vi "rwfm_AcqRead(Wfm).vi"(6 "Timeout (s)":dbl=5.0, 7 "Poll Time (ms)":u32=10, 8 "error in":errorcluster, 9 "Samps Read per Chan":i32, 10 "Sampling Info":T2={"Number of Channels"=4, "Sampling Rate"=5120.0, "Channels"=[], "Units"=[], "Offsets"=[]}, 11 "Dynamic FPGA VI Reference":T1) -> (0 "error out":errorcluster, 1 "Samples Remaining":u32, 2 "Wfm Data":waveform(sgl)[](array[waveform]), 3 "Dynamic FPGA VI Reference":T1, 4 "Data Rate [S/s]":u32, 5 "Time Stamp":timestamp)   [LabVIEW 2017, in "cRIOWfmLib.lvlib"]
doc: "Reads waveform data from the DMA FIFO."
uses:
  <vilib>/addons/InsightCM/Devices/Shared/Cms/cRIOWfmAcq/cRIOWfmLib.lvlib
  <vilib>/addons/InsightCM/Devices/Shared/Cms/cRIOWfmAcq/subVIs/RIO Wfm Cust Ctrls/rwfm_SamplingInfo.ctl
  <vilib>/addons/InsightCM/Devices/Shared/Cms/cRIOWfmAcq/subVIs/RIO Wfm Cust Ctrls/rwfm_DynamicFPGAref2.ctl
  <vilib>/Utility/error.llb/Error Cluster From Error Code.vi
  <vilib>/rvi/errors/niLvFpgaAdjustHostInterfaceError.vi
  <vilib>/rvi/interface/nirviReadWriteControl/nirviReadWriteControl.xnode
  <vilib>/rvi/interface/nirviMethod/nirviMethod.xnode
  NiFpgaLv.dll
  <vilib>/rvi/interface/Simulation/niFpgaSimulationCallBeginRW.vi
  <vilib>/FPGAPlugInAG/Dynamic/niLvFpga_ReadFifo_Dynamic.vi
  <vilib>/rvi/errors/niLvFpgaMergeErrorWithErrorCode.vi
panel:
  out "Read Time (ms)":u32
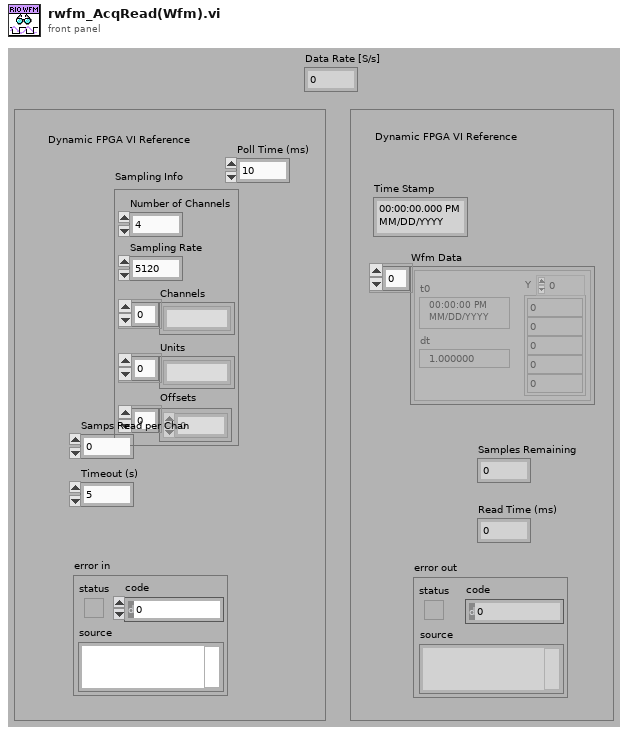
[diagram p1: front panel]
types:
  T1 = typedef "cRIOWfmLib.lvlib/rwfm_DynamicFPGAref2.ctl" = refnum<k20>
  T2 = typedef "cRIOWfmLib.lvlib/rwfm_SamplingInfo.ctl" = cluster{"Number of Channels":i32, "Sampling Rate":dbl, "Channels":string[], "Units":string[], "Offsets":sgl[]}
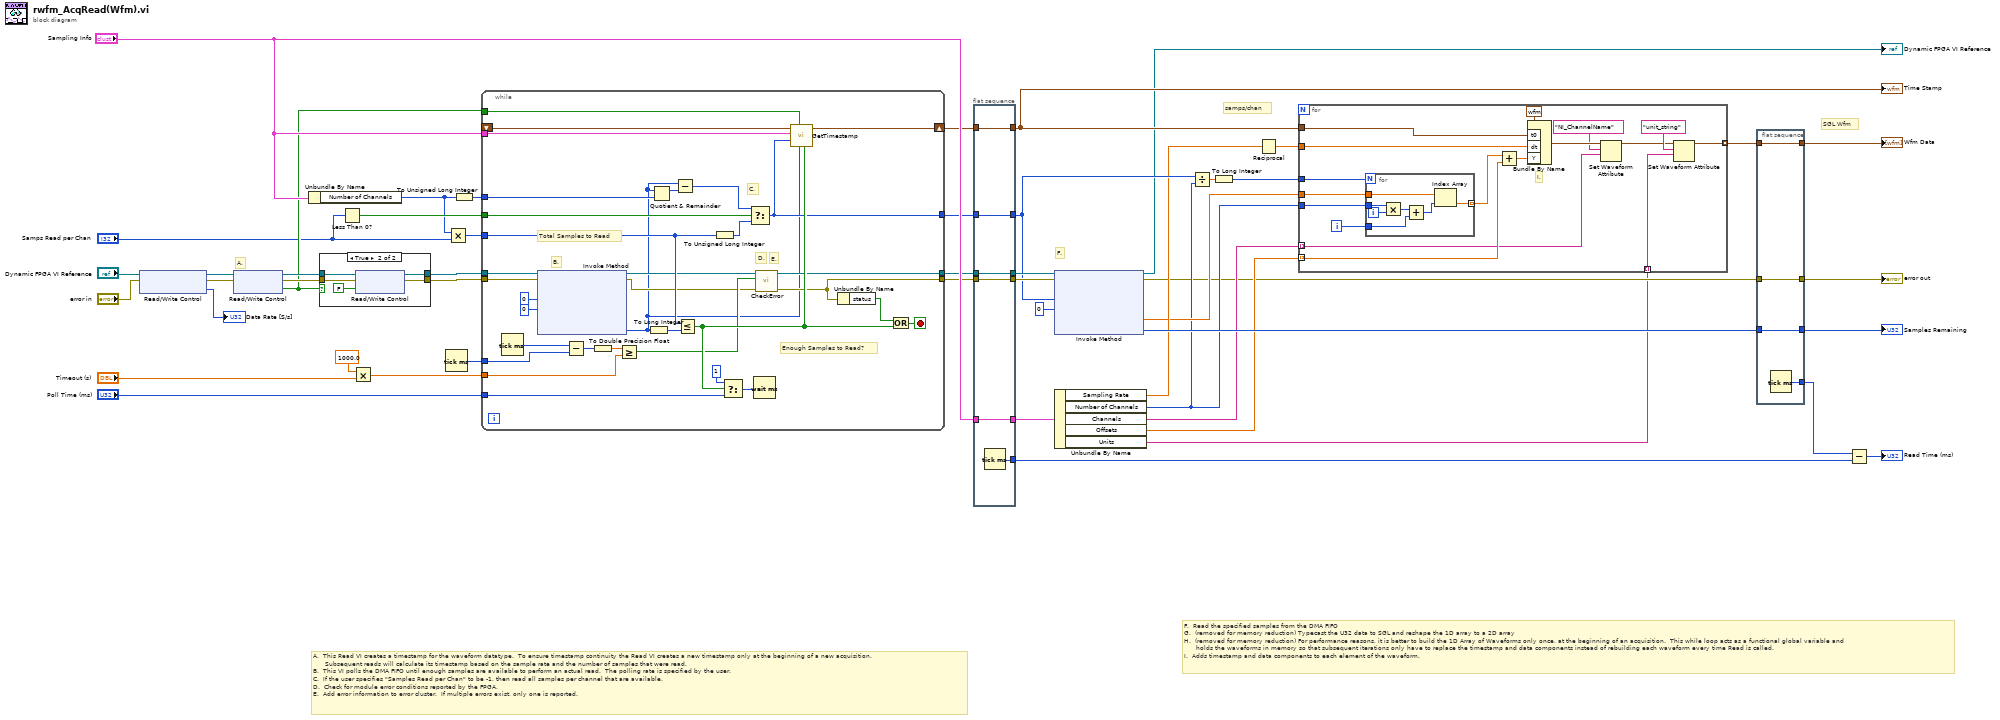
[diagram p0: block diagram]
diagram:
  # "samps/chan"
  # "SGL Wfm"
  # "F."
  # "F.  Read the specified samples from the DMA FIFO\nG.  (removed for memory reduction) Typecast the U32 data to SGL and reshape the 1D array to a 2D array\nH.  (removed for memory reduction) For performance reasons, it is better to build the 1D Array of Waveforms only once, at the beginning of an acquisition.  This while loop acts as a functional global variable and\n      holds the waveforms in memory so that subsequent iterations only have to replace the timestamp and data components instead of rebuilding each waveform every time Read is called.\nI.  Adds timestamp and data components to each element of the waveform."
  # "A.  This Read VI creates a timestamp for the waveform datatype.  To ensure timestamp continuity the Read VI creates a new timestamp only at the beginning of a new acquisition.  \n      Subsequent reads will calculate its timestamp based on the sample rate and the number of samples that were read.\nB.  This VI polls the DMA FIFO until enough samples are available to perform an actual read.  The polling rate is specified by the user.\nC.  If the user specifies \"Samples Read per Chan\" to be -1, then read all samples per channel that are available.\nD.  Check for module error conditions reported by the FPGA.\nE.  Add error information to error cluster.  If multiple errors exist, only one is reported."
  # "A."
  n1 = xnode "Read/Write Control"("FPGA VI Reference In"="Dynamic FPGA VI Reference", "error in"="error in") -> ("FPGA VI Reference Out"=w11:T1, "error out"=w14:errorcluster, "Data Rate [S/s]"=→"Data Rate [S/s]":u32)
  n2 = xnode "Read/Write Control"("FPGA VI Reference In"=w11, "error in"=w14) -> ("FPGA VI Reference Out"=w49:T1, "error out"=w50:errorcluster, "First Read"=w23:bool)
  n3 = Unbundle By Name("Sampling Info") -> ("Number of Channels"=w17:i32)
  n4 = case shown="True" w23 {
    tunnel: w49 -> [w52 w57]
    tunnel: [w52 w56] -> w48
    tunnel: w50 -> [w51 w55]
    tunnel: [w51 w54] -> w47
    frame False {
    }
    frame True {
      n5 = xnode "Read/Write Control"("FPGA VI Reference In"=w57, "error in"=w55, "First Read"=FALSE) -> ("FPGA VI Reference Out"=w56:T1, "error out"=w54:errorcluster)
    }
  }
  n6 = Less Than 0?(x="Samps Read per Chan") -> (x < 0?=w31:bool)
  n7 = Multiply(x=1000.0 ("y"), y="Timeout (s)") -> (x*y=w43:dbl)
  n8 = Tick Count (ms)() -> (millisecond timer value=w46:u32)
  n9 = Multiply(x=w17, y="Samps Read per Chan") -> (x*y=w30:i32)
  n10 = To Unsigned Long Integer(number=w17) -> (unsigned 32bit integer=w28:u32)
  n11 = while {
    tunnel: [w61] -> w34
    tunnel: [w64] -> w35
    tunnel: w23 -> [w80]
    tunnel: w48 -> [w84]
    tunnel: w47 -> [w83]
    shift-right: [w74] -> w33
    shift-left: _ -> [w81]
    tunnel: "Sampling Info" -> [w82]
    tunnel: w46 -> [w85]
    tunnel: w43 -> [w86]
    tunnel: "Poll Time (ms)" -> [w76]
    tunnel: w30 -> [w69]
    tunnel: [w67] -> w32
    tunnel: w31 -> [w72]
    tunnel: w28 -> [w68]
    stop <- w87 stop-if-true
    # "E."
    # "D."
    # "C."
    # "B."
    # "Total Samples to Read"
    # "Enough Samples to Read?"
    n12 = Tick Count (ms)() -> (millisecond timer value=w79:u32)
    n13 = xnode "Invoke Method"("FPGA VI Reference In"=w84, "error in"=w83, "Number of Elements"=u32 0, "Timeout (ms)"=0) -> ("FPGA VI Reference Out"=w63:T1, "error out"=w62:errorcluster, "Elements Remaining"=w58:u32)  [unwired: 1 out]
    n14 = Subtract(x=w79, y=w85) -> (x-y=w90:u32)
    n15 = To Double Precision Float(number=w90) -> (double precision float=w89:dbl)
    n16 = Greater Or Equal?(x=w89, y=w86) -> (x >= y?=w73:bool)
    n17 = To Long Integer(number=w58) -> (32bit integer=w71:i32)
    n18 = Quotient & Remainder(x=w58, y=w68) -> (x-y*floor(x/y)=w66:u32)  [unwired: 1 out]
    n19 = Subtract(x=w58, y=w66) -> (x-y=w65:u32)
    n20 = Less Or Equal?(x=w69, y=w71) -> (x <= y?=w78:bool)
    n21 = To Unsigned Long Integer(number=w69) -> (unsigned 32bit integer=w70:u32)
    n22 = Select(t=u32 1, s=w78, f=w76) -> (s? t:f=w77:u32)
    n23 = Select(t=w65, s=w72, f=w70) -> (s? t:f=w67:u32)
    n24 = Wait (ms)(milliseconds to wait=w77) -> ()  [unwired: 1 out]
    n25 = call <vilib>:"CheckError.vi"("error in (no error)"=w62, "timeout?"=w73, "dynamic fgpa vi reference in"=w63) -> ("error out"=w61:errorcluster, "dynamic fpga vi reference out"=w64:T1)  [unwired: 7 in]
    n26 = call <vilib>:"GetTimestamp.vi"("Enough Samples to Read"=w78, "Elements Remaining"=w58, "First Read"=w80, "Samples to Read"=w67, "Sampling Info"=w82, "Time Stamp in"=w81) -> ("Time Stamp out"=w74:timestamp)  [unwired: 5 in]
    n27 = Unbundle By Name(w61) -> ("status"=w88:bool)
    n28 = Or(x=w88, y=w78) -> (x .or. y?=w87:bool)
  }
  n29 = flat-sequence {
    tunnel: [w96] -> w15
    tunnel: "Sampling Info" -> [w95]
    tunnel: [w95] -> w37
    tunnel: [w94] -> w25
    tunnel: w35 -> [w94]
    tunnel: [w93] -> w24
    tunnel: w34 -> [w93]
    tunnel: [w92] -> w19
    tunnel: w33 -> [w92]
    tunnel: [w91] -> w22
    tunnel: w32 -> [w91]
    frame #0 {
      n30 = Tick Count (ms)() -> (millisecond timer value=w96:u32)
    }
  }
  n31 = xnode "Invoke Method"("FPGA VI Reference In"=w25, "error in"=w24, "Number of Elements"=w22, "Timeout (ms)"=0) -> ("FPGA VI Reference Out"=→"Dynamic FPGA VI Reference":T1, "error out"=w2:errorcluster, "Data"=w5:sgl[], "Elements Remaining"=w20:u32)
  n32 = Unbundle By Name(w37) -> ("Sampling Rate"=w7:dbl, "Number of Channels"=w4:i32, "Channels"=w8:string[], "Offsets"=w9:sgl[], "Units"=w1:string[])
  n33 = Divide(x=w22, y=w4) -> (x/y=w27:dbl)
  n34 = To Long Integer(number=w27) -> (32bit integer=w3:i32)
  n35 = Reciprocal(x=w7) -> (1/x=w6:dbl)
  n36 = for {
    tunnel: w19 -> [w101]
    tunnel: [w98] -> w26 mode=indexing
    tunnel: w9 -> [w112] mode=indexing
    tunnel: w8 -> [w110] mode=indexing
    tunnel: w6 -> [w102]
    tunnel: w5 -> [w107]
    tunnel: w4 -> [w106]
    tunnel: w3 -> [w103]
    tunnel: w1 -> [w97] mode=indexing
    i -> [w105]
    # "I."
    n37 = for {
      N: w103 -> [_]
      tunnel: w107 -> [w120]
      tunnel: w106 -> [w118]
      tunnel: w105 -> [w116]
      tunnel: [w114] -> w104 mode=indexing
      i -> [w119]
      n38 = Multiply(x=w118, y=w119) -> (x*y=w117:i32)
      n39 = Add(x=w117, y=w116) -> (x+y=w115:i32)
      n40 = Index Array(array=w120, index=w115) -> (element=w114:sgl)
    }
    n41 = Add(x=w104, y=w112) -> (x+y=w113:sgl[])
    n42 = Bundle By Name(cluster=waveform(sgl) {"t0"=timestamp(0 s since 1904-01-01), "dt"=1.0, "Y"=[]} ("waveform"), "t0"=w101, "dt"=w102, "Y"=w113) -> (w111:waveform(sgl))
    n43 = Set Waveform Attribute(5:w110, 6:"NI_ChannelName" ("name"), 7:w111) -> (3:w99:waveform(sgl))  [unwired: 1 in, 2 out]
    n44 = Set Waveform Attribute(5:w97, 6:"unit_string" ("name"), 7:w99) -> (3:w98:waveform(sgl))  [unwired: 1 in, 2 out]
  }
  n45 = flat-sequence {
    tunnel: [w124] -> w41
    tunnel: w2 -> [w124]
    tunnel: [w123] -> w38
    tunnel: w26 -> [w123]
    tunnel: [w122] -> w40
    tunnel: [w121] -> w29
    tunnel: w20 -> [w121]
    frame #0 {
      n46 = Tick Count (ms)() -> (millisecond timer value=w122:u32)
    }
  }
  n47 = Subtract(x=w40, y=w15) -> (x-y=→"Read Time (ms)":u32)
  "error out" <- w41
  "Samples Remaining" <- w29
  "Wfm Data" <- w38
  "Time Stamp" <- w19
